vi "PropiedadesVI.vi"() -> ()   [LabVIEW 2020]
panel:
  out "Indicador":sgl[](array[numeric])
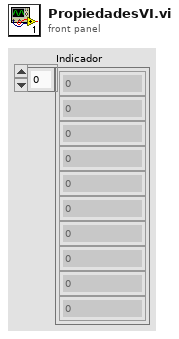
[diagram p1: front panel]
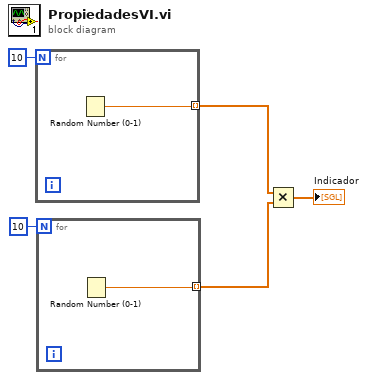
[diagram p0: block diagram]
diagram:
  n1 = for {
    N: 10 -> [_]
    tunnel: [w6] -> w2 mode=indexing
    n2 = Random Number (0-1)() -> (number: 0 to 1=w6:dbl)
  }
  n3 = for {
    N: 10 -> [_]
    tunnel: [w7] -> w3 mode=indexing
    n4 = Random Number (0-1)() -> (number: 0 to 1=w7:dbl)
  }
  n5 = Multiply(x=w2, y=w3) -> (x*y=→"Indicador":dbl[])
